vi "OCV Histogram gRPC.vi"() -> (1 "mean values of channels":dbl[](array[numeric]), 2 "std dev":dbl, 3 "range":dbl)   [LabVIEW 2019] (continued)
  n11 = Array Size(array=w20) -> (size(s)=w41:i32)
  n12 = Array Size(array=w19) -> (size(s)=w39:i32)
  n13 = Array Size(array=w14) -> (size(s)=w17:i32)
  n14 = call <vilib>:"Histogram.vi"("intervals"=w18, "X"=w22) -> ("Histogram Graph"=w32:T3)  [unwired: 6 in, 3 out]
  "Histogram Graph ch0" <- w32
  n15 = call <vilib>:"Histogram.vi"("intervals"=w18, "X"=w21) -> ("Histogram Graph"=w31:T3)  [unwired: 6 in, 3 out]
  "Histogram Graph ch1" <- w31
  n16 = call <vilib>:"Histogram.vi"("intervals"=w18, "X"=w20) -> ("Histogram Graph"=w30:T3)  [unwired: 6 in, 3 out]
  "Histogram Graph ch2" <- w30
  n17 = call <vilib>:"Histogram.vi"("intervals"=w18, "X"=w19) -> ("Histogram Graph"=w29:T3)  [unwired: 6 in, 3 out]
  "Histogram Graph ch3" <- w29
  n18 = call <vilib>:"Histogram.vi"("intervals"=w18, "X"=w14) -> ("Histogram Graph"=w13:T3)  [unwired: 6 in, 3 out]
  "Histogram Graph ch4" <- w13
  n19 = call <vilib>:"Std Deviation and Variance.vi"("X"=w22, "Weighting (Sample)"=w45) -> ("mean"=w28:dbl, "standard deviation"=w27:dbl)  [unwired: 1 out]
  "ch0 mean" <- w28
  "ch0 std dev" <- w27
  n20 = call <vilib>:"Measures of Spread.vi"("type"=w44, "x array"=w22) -> ("spread value"=w26:dbl)  [unwired: 8 in, 1 out]
  "ch0 range" <- w26
  n21 = call <vilib>:"Std Deviation and Variance.vi"("X"=w21, "Weighting (Sample)"=w43) -> ("mean"=w25:dbl, "standard deviation"=w24:dbl)  [unwired: 1 out]
  "ch1 mean" <- w25
  "ch1 std dev" <- w24
  n22 = call <vilib>:"Measures of Spread.vi"("type"=w42, "x array"=w21) -> ("spread value"=w23:dbl)  [unwired: 8 in, 1 out]
  "ch1 range" <- w23
  n23 = call <vilib>:"Std Deviation and Variance.vi"("X"=w20, "Weighting (Sample)"=w41) -> ("mean"=w11:dbl, "standard deviation"=w9:dbl)  [unwired: 1 out]
  "ch2 mean" <- w11
  "ch2 std dev" <- w9
  n24 = call <vilib>:"Measures of Spread.vi"("type"=w40, "x array"=w20) -> ("spread value"=w5:dbl)  [unwired: 8 in, 1 out]
  "ch2 range" <- w5
  n25 = call <vilib>:"Std Deviation and Variance.vi"("X"=w19, "Weighting (Sample)"=w39) -> ("mean"=w10:dbl, "standard deviation"=w8:dbl)  [unwired: 1 out]
  "ch3 mean" <- w10
  "ch3 std dev" <- w8
  n26 = call <vilib>:"Measures of Spread.vi"("type"=w38, "x array"=w19) -> ("spread value"=w4:dbl)  [unwired: 8 in, 1 out]
  "ch3 range" <- w4
  n27 = call <vilib>:"Std Deviation and Variance.vi"("X"=w14, "Weighting (Sample)"=w17) -> ("mean"=w6:dbl, "standard deviation"=w7:dbl)  [unwired: 1 out]
  "ch4 mean" <- w6
  "ch4 std dev" <- w7
  n28 = call <vilib>:"Measures of Spread.vi"("type"=w16, "x array"=w14) -> ("spread value"=w3:dbl)  [unwired: 8 in, 1 out]
  "ch4 range" <- w3
  n29 = Build Array(w28, w25, w11, w10, w6) -> (→"mean values of channels":dbl[])
  n30 = Build Array(w27, w24, w9, w8, w7) -> (w36:dbl[])
  n31 = call-poly <vilib>:"Mean.vi"("X"=w36) -> ("mean"=→"std dev":dbl)  [unwired: 1 out]
  n32 = Build Array(w26, w23, w5, w4, w3) -> (w34:dbl[])
  n33 = call-poly <vilib>:"Mean.vi"("X"=w34) -> ("mean"=→"range":dbl)  [unwired: 1 out]
  n34 = Bundle By Name(cluster="Results Cluster", "Waveform Chart ch0"=w22, "Waveform Chart ch1"=w21, "Waveform Chart ch2"=w20, "Waveform Chart ch3"=w19, "Waveform Chart ch4"=w14, "Histogram Graph ch0"=w32, "Histogram Graph ch1"=w31, "Histogram Graph ch2"=w30, "Histogram Graph ch3"=w29, "Histogram Graph ch4"=w13, "ch0 mean"=w28, "ch0 std dev"=w27, "ch0 range"=w26, "ch1 mean"=w25, "ch1 std dev"=w24, "ch1 range"=w23, "ch2 mean"=w11, "ch2 std dev"=w9, "ch2 range"=w5, "ch3 mean"=w10, "ch3 std dev"=w8, "ch3 range"=w4, "ch4 mean"=w6, "ch4 std dev"=w7, "ch4 range"=w3) -> (→"Results Cluster":T4)
